vi "Project_and_Plugin Template Creation.vi"(0 "Project Path":path, 5 "Description":string, 11 "error in (no error)":errorcluster) -> (15 "error out":errorcluster)   [LabVIEW 2021, in "Converter.lvlib"]
uses:
  Converter.lvlib
  Measurement Plugin Generator/_Editor/MeasurementService Editor.lvlib
  Path Functions/Path Functions.lvlib
  Converter Reusables/Converter Reusables.lvlib
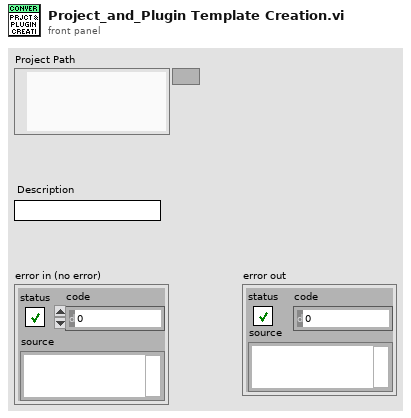
[diagram p1: front panel]
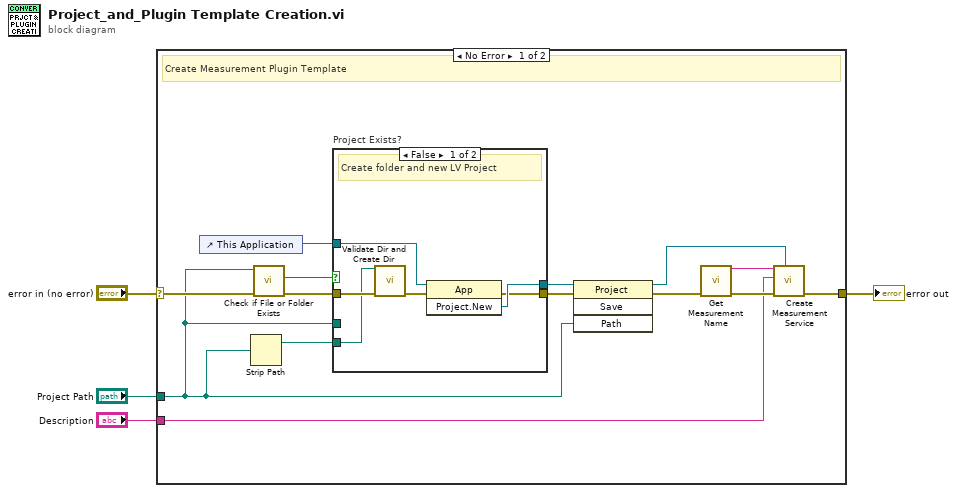
[diagram p0: block diagram]
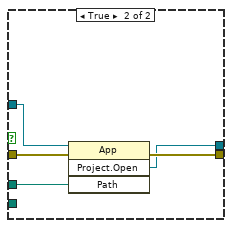
[diagram p2: hidden frame]
diagram:
  n1 = case shown="No Error" "error in (no error)" {
    selector: "error in (no error)" -> [w17 w30]
    tunnel: "Project Path" -> [w14 _]
    tunnel: [w5 w30] -> w2
    tunnel: "Description" -> [w9 _]
    frame No Error {
      # "Create Measurement Plugin Template"
      n2 = control-ref of="This Application"() -> (w13:refnum<vi>)
      n3 = Strip Path(path=w14) -> (stripped path=w18:path)  [unwired: 1 out]
      n4 = call <vilib>:"Check if File or Folder Exists.vi"("error in (no error)"=w17, "path"=w14) -> ("error out"=w16:errorcluster, "file or folder exists?"=w15:bool)  [unwired: 7 in, 1 out]
      n5 = case "Project Exists?" shown="False" w15 {
        tunnel: [w24 w26] -> w8
        tunnel: [w23 w27] -> w7
        tunnel: w18 -> [w20 _]
        tunnel: w16 -> [w21 w29]
        tunnel: w14 -> [_ w28]
        tunnel: w13 -> [w22 w25]
        frame False {
          # "Create folder and new LV Project"
          n6 = call "Validate Dir and Create Dir.vi"("Directory"=w20, "error in (no error)"=w21) -> ("error out"=w19:errorcluster)  [unwired: 12 in, 1 out]
          n7 = invoke class="App" method="Project.New"(reference=w22, error in=w19) -> (error out=w23:errorcluster, "Project:New"=w24:refnum<vi>)  [unwired: 1 in, 1 out]
        }
        frame True {
          n8 = invoke class="App" method="Project.Open"(reference=w25, error in=w29, "Path"=w28) -> (error out=w27:errorcluster, "Project:Open"=w26:refnum<vi>)  [unwired: 1 in, 2 out]
        }
      }
      n9 = invoke class="Project" method="Save"(reference=w8, error in=w7, "Path"=w14) -> (reference out=w12:refnum<vi>, error out=w6:errorcluster)  [unwired: 1 in, 2 out]
      n10 = call "Get Measurement Name.vi"("error in (no error)"=w6) -> ("Name Out"=w10:string, "error out"=w11:errorcluster)  [unwired: 13 in]
      n11 = call "Create Measurement Service.vi"("project ref"=w12, "error in (no error)"=w11, "measurement plug-in description"=w9, "measurement plug-in name"=w10) -> ("error out"=w5:errorcluster)  [unwired: 7 in]
    }
    frame Error {
    }
  }
  "error out" <- w2
